vi "AlliGator Update Phasor Plot Image v2.vi"(5 "Image Control Refnum":T1 caption="Phasor Plot Display Refnum", 7 "Phasor Plot Color Scale":refnum<vi>, 8 "Error In":errorcluster, 9 "Phasor Plot Image Elements to Update":string[](array[string]), 10 "AlliGator Internal Variables DVR":refnum<data-value>, 11 "Phasor Plot Display Range Refnum":refnum<vi>) -> (0 "Error Out":errorcluster, 1 "Message":string, 2 "AlliGator Internal Variables DVR":refnum<data-value>)   [LabVIEW 2021, in "AlliGator Phasor Plot.lvlib"]
doc: "Updates the Phasor Plot image including its overlays."
uses:
  AlliGator Phasor Plot.lvlib
  Internal Variables/AlliGator Internal Variables v2.ctl
  <vilib>/vision/Image Controls.llb/IMAQ Image.ctl
  Internal Variables/AlliGator Gate Image Set.ctl
  Files/AlliGator FLI Dataset Type.ctl
  Files/AlliGator Data Series Type.ctl
  Dual-Channel Datasets/AlliGator Dataset Channel.ctl
  Settings/AlliGator Gate Arithmetic.ctl
  Source Image/AlliGator Displayed Image.ctl
  Image/Named ROI Description.ctl
  Phasor Graph/AlliGator Decay Metadata v3.ctl
  Decay Analysis/Decay Preprocessing/AlliGator Decay Background Subtraction Info.ctl
  Decay Analysis/Decay Preprocessing/AlliGator Baseline Subtraction Method.ctl
  Graphs/XY Graph/XY Graph Plot Shift Parameters.ctl
  Graphs/XY Graph/XY Graph Plot Shift Method.ctl
  Decay Analysis/Decay Preprocessing/AlliGator Decay Extrapolation Parameters.ctl
  Phasor/Calibration Phasor (m, phi).ctl
  Phasor/Phasor Reference Series.ctl
  Phasor/Phasor Calibration Map v2.ctl
  Phasor/Phasor (g, s).ctl
  Phasor Graph/AlliGator Raw Phasor Plot Data v5.ctl
  Phasor/Phasor Standard Deviation Options.ctl
  AlliGator Phasor Multi-Harmonic Data.ctl
  Phasor/Phasor Harmonic Data.ctl
  Decay Fit Parameter Map/AlliGator Decay Fit Options & Parameters v4.ctl
  Fits/IRF(X)PSED/Decay Fit Options v4.ctl
  Fits/Decay Convolution/Decay Model.ctl
  Fits/Residual Type.ctl
  Fits/IRF(X)PSED/Fit Weights Type v2.ctl
  Fits/Non-linear Fitting Method v2.ctl
  Fits/Fit Calculation Method.ctl
  Fits/Non-linear Fitting Algorithm.ctl
  Decay Analysis/Decay Fit/AlliGator Decay Fit Parameter Constraints 2.ctl
  Fits/IRF(X)PSED/Decay Fit Parameters In List.ctl
  Fits/IRF(X)PSED/MLE Baseline Offset Type.ctl
  Decay Analysis/Decay Preprocessing/AlliGator Decay Preprocessing Parameters.ctl
  Fits/IRF(X)PSED/Decay Fit Parameters & Derived Quantities List v2.ctl
  Fits/IRF(X)PSED/Decay Fit Result Constraint.ctl
  Decay Fit Parameter Map/AlliGator Parameter Maps Data.ctl
  Image/Image Control Refnum.ctl
  Globals, Variables, Constants/AlliGator Variables List.ctl
  a24687bc-c119-402d-9a1a-602e9bf75a15.vi
  Variant/Variant to Data/Variant to U16.vi
  Phasor Calibration/AlliGator Phasor Calibration.lvlib
  GUI/AlliGator GUI.lvlib
  Settings/AlliGator Settings.lvlib
  Time/Time.lvlib
  Globals, Variables, Constants/AlliGator Globals, Variables & Constants.lvlib
  Variant/Variant to Data/Variant to Data.lvlib
  Phasor/Phasor.lvlib
  7bec4d3f-1ec9-40da-bd4c-cfd082c5c359.vi
  Image/Image.lvlib
  Decay Analysis/Decay Preprocessing/AlliGator Decay Preprocessing.lvlib
  Graphs/XY Graph/XY Graph Add-Ons.lvlib
  Phasor Graph/AlliGator Phasor Graph.lvlib
  Files/AlliGator Files.lvlib
  Internal Variables/AlliGator Internal Variables.lvlib
  Source Image/AlliGator Source Image.lvlib
  Fits/Fits.lvlib
  Decay Analysis/Decay Fit/AlliGator Decay Fit.lvlib
  Dual-Channel Datasets/AlliGator Dual-Channel Datasets.lvlib
  Decay Fit Parameter Map/AlliGator Decay Fit Parameter Map.lvlib
panel:
  out "CPU (s)":dbl
  # "see the AlliGator License on the block diagram (Ctrl+E or Window:Show Block Diagram)"
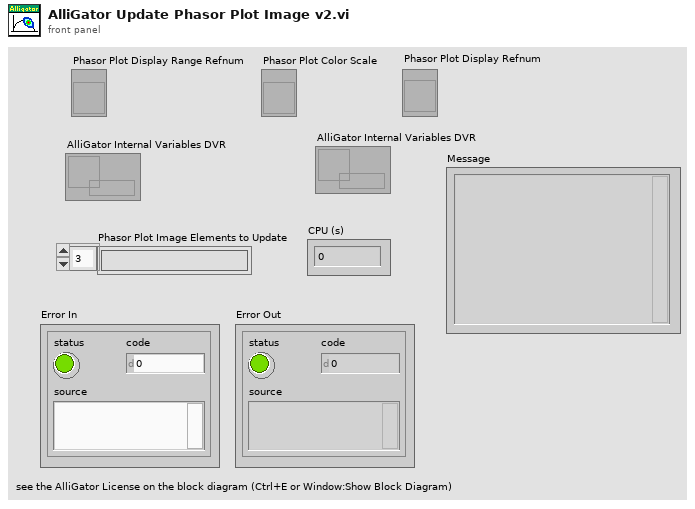
[diagram p1: front panel]
types:
  T1 = typedef "Image.lvlib/Image Control Refnum.ctl" = refnum<vi>
  T2 = typedef "AlliGator Globals, Variables & Constants.lvlib/AlliGator Variables List.ctl" = enum16{"---- GUI ----", "GUI:Initialization Status", "GUI:State Indicators Refnum", "GUI:Original AlliGator Menu Items", "GUI:Current Action Loop State", "GUI:Script in progress", "GUI:Playback", "GUI:Loop Playback", "GUI:Search ROI Used", "GUI:Search ROI", "Decay Graph Max Legend Size", "Intensity Graph Max Legend Size", "Decay Statistics Graph Max Legend Size", "Phasor Graph Max Legend Size", "Phasor Ratio Graph Max Legend Size", "Lifetime Graph Max Legend Size", "---- Files ----", "Files:Export Dataset Frames as Individual Files", "Files:Show Batch Export Help Balloons", "Files:Frames in Dataset", "Files:ptu File Frame Start Indices", "Files:Current Frame in Dataset", "Files:Current Frame Timestamp", "Files:Dataset Loaded", "Files:Dataset Metadata", "Files:Dataset Channel", "Files:Dataset Data Description", "Files:Background Dataset Metadata", "Files:Background Dataset Channel", "Files:Background Dataset Data Description", "Files:Background File Subtraction", "Files:Background File Path", "Files:Background File Pile-up Correction", "Files:Background File Pixel Well Capacity", "Files:Background File Scaling Factor", "Files:Current Dataset Load Settings", "Files:Dataset Path", "Files:ICCD-specific Information", "Files:Macrotime Gate Separation", "------ Python Plugins ------", "Python Plugins:Information", "Python Plugins:Python Session", "Python Plugins:Valid Python Session?", "---- Source Image ----", "Source Image:ROIs", "Source Image:Current ROI", "Source Image:ROI Event Refnum", "X_Source Image:Display Range", "X_Source Image:Palette Information", "X_Source Image:Type of Displayed Image", "X_Time Gate Slider", "Source Image:Palette List", "Source Image:Scale", "Source Image:ROI Overlay Color", "Source Image:Overlay to Erase", "Source Image:Is Displayed Image Accumulated", "Source Image:White Light Image Modified", "Source Image:Mask Image Modified", "---- Image Profile Window ----", "Image Profile:Window Event Refnum", "Image Profile:IntensityType", "Image Profile:Intensity Average Type", "Image Profile:Intensity-weighted SDV", "Image Profile:Box Profile Type", "Image Profile:Window Open", "Image Profile:Plotted Fit Parameter", "------ Phasor Graph -------", "Phasor Graph:Show Line", "---- Phasor Plot ---", "Phasor Plot:Parameters Changed", "Phasor Plot:FLI Dataset Modified since last Calculation", "Phasor Harmonics Data", "Selected Phasor Harmonics", "Phasor Harmonic Manager Event Refnum", "Phasor Plot:ROIs", "Phasor Plot:Current ROI", "Phasor Plot:ROI Event Refnum", "Phasor Plot:Image Reference Points", "Phasor Plot:Computed", "Phasor Plot:Palette Information", "Phasor Plot:Palette List", "Phasor Plot:Phasor Ratio Palette Information", "Phasor Plot:Phasor Ratio Palette List", "Phasor Plot:Image Scale", "Phasor Plot:Image Overlay to Erase", "Phasor Plot:Image Elements to Update", "Phasor Plot:Current Calculation Parameters", "Phasor Plot:Current Calibration Options", "Phasor Plot:Reset Cumulated Phasor Plot", "Phasor Plot:Reference 1", "Phasor Plot:Lifetime Reference 1", "Phasor Plot:Reference 1 Frequency", "Phasor Plot:Reference 2", "Phasor Plot:Lifetime Reference 2", "Phasor Plot:Reference 2 Frequency", "---- Decay Analysis ----", "Number of Selected Decays to Fit", "LS Fit Results", "LAR Fit Results", "BS Fit Results", "Last Decay Max - Min", "Best Fit Parameters", "Best Fit Parameter Names", "Actual Size X", "Actual Size Y", "Binning X", "Binning Y", "Actual # Gates", "Dataset Number", "Gates to...", "Gates Skipped", "Gates to keep", "Gate Step", "Gate Separation", "Reversed Gates", "Pile-up Correction", "Pixel Well Capacity", "Background Subtracted", "Background Subtraction Method", "Background Definition Range", "Background File (deprecated)", "Number of Dataset Accumulated", "Array of Accumulated Dataset Paths", "Do Averaged Datasets", "Destination File Path", "Process Plot Target", "Use 1/D as Phasor Frequency", "---- Decay Fit Parameter Map -----", "Decay Fit Parameter Map:Palette Information", "Decay Fit Parameter Map:Palette List", "Decay Fit Parameter Map:X Resolution", "Decay Fit Parameter Map:Y Resolution", "Decay Fit Parameter Map:Use Decay Fit Result Constraints", "Decay Fit Parameter Map:Decay Fit Result Constraints", "Decay Fit Parameter Map:Decay Fit Result Constraints Applied", "---- Parameter Map ----", "Parameter Map:Palette Information", "Parameter Map:Palette List", "------- Local Decay Window ---------", "Local Decay Graph Window:Event Refnum", "Local Decay Graph Window:Use normalized IRF for convolution", "----- Miscellaneous ----", "Misc:Skippable Dialog Windows Status"}
  T3 = typedef "AlliGator Internal Variables.lvlib/AlliGator Internal Variables v2.ctl" = cluster{"----------------------------- Images -----------------------------":u8, "Displayed Image":T4, "White Light Image":T4, "Mask Image":T4, "ROI Mask Image":T4, "Current Dataset Images 1":T5, "Background Dataset Images 1":T5, "Current Dataset Images 2":T5, "Background Dataset Images 2":T5, "Current Dataset Arithmetic Images":T5, "Accumulated Dataset Images 1":T5, "Accumulated Dataset Images 2":T5, "Accumulated Dataset Arithmetic Images":T5, "----------------------------- File Paths -----------------------------":u8, "Phasor Plot Image":T4, "Decay Fit Parameter Map Image":T4, "Parameter Map Image":T4, "Single Data Point Path":path, "White Light Image Path":path, "Mask Image Path":path, "Time-Series Folder":path, "[Time-Series Paths]":path[], "----------------------------- FLI Dataset -----------------------------":u8, "Current Dataset":i32, "Single Dataset Type":T6, "Current Folder":string, "AlliGator Data Series Type":T7, "# Datasets":i32, "Dual-Channel Dataset":bool, "Selected Channel Name":string, "Dataset Channel":T8, "Channel Arithmetic":T9, "Dual-Channel Background Dataset":bool, "Background Channel":T8, "Dual-Channel Accumulated Dataset":bool, "Start Time":dbl, "[Time-Series Timestamps]":dbl[], "[Intensity Corrections]":dbl[], "Time Series Script":bool, "Type of Displayed Image":T10, "Gate Image Slide":u16, "# Gates":i32, "ROIs":T11[], "----------------------------- Decays -----------------------------":u8, "ROI Decay":cluster{"t Array":dbl[], "I Array":dbl[]}, "Valid Decay":bool, "Decay  Metadata":T13, "Reference Decay Plot Name":string, "Reference Decay":cluster{"t Array":dbl[], "I Array":dbl[]}, "Decay Shift Plot":cluster{"Time Stamps":dbl[], "Decay Shifts":dbl[]}, "[Decays Max Values]":sgl[], "[Decays Min Values]":sgl[], "----------------------------- Calibration -----------------------------":u8, "Calibration Phasor":T19, "Calibration Phasor Series":T20, "Phasor Calibration Map":T21, "Calibration Map MD5 Digest":string, "----------------------------- Phasor Graph -----------------------------":u8, "Last Raw Phasor":T22, "Last Calibrated Phasor":T22, "Last Calibrated Phasor SDV":T22, "Phasor Graph:Phasor Plot":cluster{"g Array":dbl[], "s Array":dbl[]}, "Phasor Graph:Phasor SDV Plot":cluster{"g Array":dbl[], "s Array":dbl[]}, "[Phasor Graph:Raw Phasor Plots]":T23[], "Phasor Plot locked to Ref 1":i32, "[Phasor Plot(s) locked to Ref 1]":i32[], "[Phasor Plot(s) locked to Ref 2]":i32[], "[Pixel Phasors]":T22[], "----------------------------- Phasor Plot -----------------------------":u8, "[[Sum Image]]":dbl[][], "[[CSG Phasors]]":csg[][], "[[Valid Pixel?]]":bool[][], "[[Phasor Ratios]]":dbl[][], "[[Average Lifetimes]]":dbl[][], "Amplitude Weighted Average Lifetime":bool, "I/m/phi Dataset":cluster{"I/m/phi Dataset?":bool, "Base Frequency":dbl[unit], "Harmonic Orders":u8[]}, "Multi Phasor Plot Data":T25, "----------------------------- Decay Fit Parameter Map -----------------------------":u8, "Decay Fit Options & Parameters":T27, "Fit Options: Decay Preprocessing Parameters":T38, "Fit Options: Reference Decay":cluster{"t Array":dbl[], "I Array":dbl[]}, "Is Full Image Parameters Map":bool, "Is Single-Pixels Parameters Map":bool, "NLSF Parameters Map X Resolution":i32, "NLSF Parameters Map Y Resolution":i32, "[Single Decay Fit Parameters]":dbl[], "Fit Model":T29, "[[Multiple Decays Fit Parameters]]":dbl[][], "[[Multiple Decays Fit Parameter SDVs]]":dbl[][], "[[IRFs]]":dbl[][], "[ROI Descriptors]":T12[], "IRF Array Time Axis":dbl[], "Decay Array Time Axis":dbl[], "[Decay Fit Parameter Names]":T39[], "[Decay Sum]":dbl[], "Array of Decay Fit Result Constraints":T40[], "Selected ROIs Array":bool[], "----------------------------- Parameter Maps -----------------------------":u8, "[Map Set Names]":string[], "[Parameter Maps]":T41[], "[[User-defined Quantities]]":dbl[][], "User-defined Quantity":string}
  T4 = typedef "IMAQ Image.ctl" = refnum<image>
  T5 = typedef "AlliGator Internal Variables.lvlib/AlliGator Gate Image Set.ctl" = cluster{"SGL Gate Images":T4[], "SGL Sum Image":T4, "SGL Max Image":T4, "SGL Min Image":T4}
  T6 = typedef "AlliGator Files.lvlib/AlliGator FLI Dataset Type.ctl" = enum16{"HDF5 FLI Dataset", "Gate Image Folder", ".sdt FLI Dataset (Becker & Hickl)", ".ptu FLI Dataset (PicoQuant)", "SS1 FLI Dataset", "SS2 FLI Dataset", "I/m/phi Dataset", ".bin FLI Dataset (PicoQuant Binned)", ".bin FLI Dataset (Piccolo Binned)", ".mat FLI Dataset"}
  T7 = typedef "AlliGator Files.lvlib/AlliGator Data Series Type.ctl" = enum16{"Not a Supported Series", "Gate Images Folder Series", "SwissSPAD 2 Dataset Series", "B&H FLI Dataset Series", "PicoQuant PTU FLI Dataset Series", "PicoQuant BIN FLI Dataset Series", "Piccolo hist BIN FLI Dataset Series", "HDF5 FLI Dataset Series"}
  T8 = typedef "AlliGator Dual-Channel Datasets.lvlib/AlliGator Dataset Channel.ctl" = enum16{"G2", "INT"}
  T9 = typedef "AlliGator Settings.lvlib/AlliGator Gate Arithmetic.ctl" = enum16{"None", "INT-G2", "G2/INT*<INT>", "(1 - G2/INT)*<INT>"}
  T10 = typedef "AlliGator Source Image.lvlib/AlliGator Displayed Image.ctl" = enum16{"Single Gate", "Sum of All Gates", "Max of All Gates", "Min of All Gates", "-", "White Ligth Image", "Mask Image"}
  T11 = typedef "Image.lvlib/Named ROI Description.ctl" = cluster{"ROI Descriptor":T12, "ROI Name":string, "Overlay Color":u32}
  T12 = typedef "ROI Descriptor" = cluster{"Global Rectangle":i32[], "Contours":cluster{"ID":enum32{"External", "Internal"}, "Type":u32, "Coordinates":i32[]}[]}
  T13 = typedef "AlliGator Phasor Graph.lvlib/AlliGator Decay Metadata v3.ctl" = cluster{"ROI Descriptor":T12, "ROI Center":cluster{"X":i32, "Y":i32}, "Decay Background Subtraction Info":T14, "Decay Reverted":bool, "Decay Smoothened":bool, "Decay Straightened":bool, "Fitted Tau (Decay Straightening)":dbl, "Decay Shift Parameters":T16, "Decay Shifted":bool, "Decay Extrapolated":bool, "Decay Extrapolation Parameters":T18, "Decay Normalized":bool, "Fold Decay":bool, "# Folds":u32}
  T14 = typedef "AlliGator Decay Preprocessing.lvlib/AlliGator Decay Background Subtraction Info.ctl" = cluster{"Laser Period":dbl[unit], "Gate Duration":dbl[unit], "Baseline Subtraction Method":T15, "Background Definition Range":cluster{"Min Gate":dbl[unit], "Max Gate":dbl[unit]}, "Total Intensity w/o Bkgd Subtraction":dbl, "Bkgd-subtracted Intensity (exp)":dbl, "# Data Points":i32, "Background/Gate":dbl, "Fitted Lifetime":dbl[unit], "Bkgd-subtracted Intensity (theo)":dbl}
  T15 = typedef "AlliGator Decay Preprocessing.lvlib/AlliGator Baseline Subtraction Method.ctl" = enum16{"Mean", "Min", "Square Gated Single-Exponential", "File", "Constant"}
  T16 = typedef "XY Graph Add-Ons.lvlib/XY Graph Plot Shift Parameters.ctl" = cluster{"Type":T17, "Shift":dbl[unit], "Threshold":dbl, "Rotate":bool}
  T17 = typedef "XY Graph Add-Ons.lvlib/XY Graph Plot Shift Method.ctl" = enum16{"Default", "CFD", "Threshold", "Cross-Correlation"}
  T18 = typedef "AlliGator Decay Preprocessing.lvlib/AlliGator Decay Extrapolation Parameters.ctl" = cluster{"Additional Points":u32, "Head Fraction":dbl, "Fitted Tau":dbl, "Use Periodicity":bool, "Use Cursors":bool, "Tail Fraction":dbl}
  T19 = typedef "Phasor.lvlib/Calibration Phasor (m, phi).ctl" = cluster{"m":dbl, "phi":dbl, "Phasor Frequency":dbl[unit], "Reference Lifetime":dbl[unit]}
  T20 = typedef "Phasor.lvlib/Phasor Reference Series.ctl" = cluster{"m Array":dbl[], "phi Array":dbl[], "Phasor Frequency":dbl[unit], "Calibration Lifetime":dbl[unit]}
  T21 = typedef "Phasor.lvlib/Phasor Calibration Map v2.ctl" = cluster{"Phasor Frequency":dbl[unit], "Calibration Lifetime":dbl[unit], "ROI Centers":cluster{"X":i32, "Y":i32}[], "ROI Descriptors":T12[], "Map Resolution X":i32, "Map Resolution Y":i32, "z Array":cdb[]}
  T22 = typedef "Phasor.lvlib/Phasor (g, s).ctl" = cluster{"g":dbl, "s":dbl}
  T23 = typedef "AlliGator Phasor Graph.lvlib/AlliGator Raw Phasor Plot Data v5.ctl" = cluster{"Phasor Plot Name":string, "Raw Phasor Plot":T22[], "Phasor Frequency":dbl[unit], "[Decay Metadata]":T13[], "Raw Phasor Plot SDV":T22[], "Phasor SDV Options":T24, "[Calibration Phasor]":T19[], "Intensity Array":dbl[]}
  T24 = typedef "Phasor.lvlib/Phasor Standard Deviation Options.ctl" = cluster{"Compute Estimated SDV":bool, "# Replicas":u32, "Use Estimated Average Phasor":bool}
  T25 = typedef "AlliGator Phasor Plot.lvlib/AlliGator Phasor Multi-Harmonic Data.ctl" = cluster{"Base Frequency":dbl[unit], "# Harmonics":u8, "Harmonic Orders":u8[], "Phasor Plot Settings Checksum":u64, "Phasor Harmonic Data Array":T26[]}
  T26 = typedef "Phasor.lvlib/Phasor Harmonic Data.ctl" = cluster{"Phasor Harmonic Name":string, "Phasor Plot Settings Checksum":u64, "Phasor Frequency":dbl[unit], "Base Frequency":dbl[unit], "Harmonic Order":u8, "Phasor Plot Parameters":string, "Phasor Array [[CSG]]":csg[][], "Dataset File Path":path}
  T27 = typedef "AlliGator Decay Fit Parameter Map.lvlib/AlliGator Decay Fit Options & Parameters v4.ctl" = cluster{"SYNC Period":dbl[unit], "Fit Options":T28, "Fit Parameter Constraints":T35[], "MLE Baseline Offset":dbl, "MLE Baseline Offset Type":T37}
  T28 = typedef "Fits.lvlib/Decay Fit Options v4.ctl" = cluster{"Show Fit Residuals":bool, "Fit Model":T29, "Residual Type":T30, "Max Decay Percentile":dbl, "Min Decay Percentile":dbl, "Show Full Decay":bool, "Weights":T31, "Fitting Method":T32, "Compute Parameter Uncertainties":bool, "Periodic Boundaries":bool, "Model Calculation":T33, "Period":dbl[unit], "Termination Criteria":cluster{"Max Iterations":i32, "Max Function Calls":i32, "Max Time":dbl[unit], "Function Tolerance":dbl, "Parameter Tolerance":dbl, "Gradient Tolerance":dbl, "Min Lambda":dbl, "Max Lambda":dbl, "Initial Tick Count":u32}, "Offset Resolution":dbl[unit], "Use Local IRF":bool, "Fitting Algorithm":T34, "Show Confidence Interval ":bool, "Confidence Level":dbl}
  T29 = typedef "Fits.lvlib/Decay Model.ctl" = enum16{"1-Exponential", "2-Exponentials"}
  T30 = typedef "Fits.lvlib/Residual Type.ctl" = enum16{"Standard", "Normalized", "Reduced"}
  T31 = typedef "Fits.lvlib/Fit Weights Type v2.ctl" = enum16{"Unweighted", "1/Variance (Neyman)", "1/Variance (Pearson)", "Best of All"}
  T32 = typedef "Fits.lvlib/Non-linear Fitting Method v2.ctl" = enum16{"Least Square", "Least Absolute Residual", "Bisquare", "MLE", "-", "Best of All"}
  T33 = typedef "Fits.lvlib/Fit Calculation Method.ctl" = enum16{"Simulation", "Convolution", "Integration"}
  T34 = typedef "Fits.lvlib/Non-linear Fitting Algorithm.ctl" = enum16{"Levenberg-Marquardt", "Trust-Region Dogleg"}
  T35 = typedef "AlliGator Decay Fit.lvlib/AlliGator Decay Fit Parameter Constraints 2.ctl" = cluster{"Fit Parameter":T36, "Min Value":dbl, "Max Value":dbl, "Global":bool, "Used":bool}
  T36 = typedef "Fits.lvlib/Decay Fit Parameters In List.ctl" = enum16{"Offset", "Baseline", "A_1", "tau_1", "A_2", "tau_2"}
  T37 = typedef "Fits.lvlib/MLE Baseline Offset Type.ctl" = enum32{"Absolute", "Percentage"}
  T38 = typedef "AlliGator Decay Preprocessing.lvlib/AlliGator Decay Preprocessing Parameters.ctl" = cluster{"Background Subtraction":bool, "Straighten Decay":bool, "Reverse Gates":bool, "1-Normalized Decay":bool, "Smoothen Decay":bool, "Smoothing Parameter":dbl, "Shift Decay":bool, "Decay Shift Parameters":T16, "Extrapolate Decay":bool, "Additional Points":u32, "Head Fraction":dbl, "Pixel-Normalize Decay":bool, "Use Periodicity":bool, "Use Cursors":bool, "Tail Fraction":dbl, "Use Decay Pre-Processing":bool, "Fold Decay":bool, "# Folds":u32, "[0-1]-Normalized Decay":bool}
  T39 = typedef "Fits.lvlib/Decay Fit Parameters & Derived Quantities List v2.ctl" = enum16{"Offset", "Baseline", "A_1", "tau_1", "A_2", "tau_2", "<tau>_a", "f1_a", "f2_a", "<tau>_i", "f1_i", "f2_i", "-", "R^2", "Chi^2"}
  T40 = typedef "Fits.lvlib/Decay Fit Result Constraint.ctl" = cluster{"Fit Parameter":enum16{"Offset", "Baseline", "A_1", "tau_1", "A_2", "tau_2", "<tau>_a", "f1_a", "f2_a", "<tau>_i", "f1_i", "f2_i", "-", "R^2", "Chi^2", "Max Relative Residual", "<Residual ACF>", "Residual ACF SDV", "tau_2/tau_1"}, "Min Value":dbl, "Max Value":dbl, "Use Constraint":bool}
  T41 = typedef "AlliGator Decay Fit Parameter Map.lvlib/AlliGator Parameter Maps Data.ctl" = cluster{"Map Set Name":string, "[Parameter Names]":string[], "[[Parameters]]":dbl[][], "[[Parameter SDVs]]":dbl[][], "Decay Array Time Axis":dbl[], "[[IRFs]]":dbl[][], "IRF Array Time Axis":dbl[], "X Resolution":i32, "Y Resolution":i32, "Intensity Array":dbl[]}
  T42 = typedef "Phasor.lvlib/Phasor Calibration Type.ctl" = enum16{"None", "Single Phasor", "Phasor Series", "Phasor Map"}
  T43 = cluster{"Use Backup Calibration if needed?":bool, "Calibration Type":T42}
  T44 = typedef "AlliGator Phasor Calibration.lvlib/AlliGator Phasor Calibration Options.ctl" = cluster{"Phasor Frequency":dbl[unit], "Phasor Calibration":cluster{"Calibration Lifetime":dbl[unit], "Calibration Type":T42, "Calibration Map Algorithm":T45, "Use Backup Calibration if needed":bool, "Backup Calibration Type":enum16{"Single Calibration", "Nearest Valid Calibration"}}}
  T45 = typedef "AlliGator Phasor Calibration.lvlib/AlliGator Calibration Map Algorithm.ctl" = enum16{"Simple Search", "Min Distance"}
  T46 = typedef "AlliGator Phasor Plot.lvlib/AlliGator Phasor Plot Parameters v2.ctl" = cluster{"Phasor Frequency":dbl[unit], "Decay Preprocessing Options & Parameters":T47, "FLI Dataset Modified":bool, "Source Image Settings":cluster{"Low Count Pixels Rejection Options":T49, "High Count Pixels Rejection Options":T50}, "Data Information":cluster{"Gate Width":dbl[unit], "Gate Separation":dbl[unit], "Step (Gate Separation)":i32, "Laser Period":dbl[unit], "SYNC Period":dbl[unit], "Channel Name":u16, "Channel Arithmetic":T9, "Pile-up Correction":bool, "Pixel Well Capacity":u32, "Dataset Scaling Factor":dbl}, "Phasor Plot":cluster{"Phasor Plot Smoothing Options":T51, "Phasor Plot Size":T54, "Selected Image ROI(s)":bool, "All Image ROIs":bool, "Selected Source Image ROI":i32, "Source Image ROIs":T11[]}}
  T47 = typedef "AlliGator Decay Preprocessing.lvlib/AlliGator Decay Preprocessing Options.ctl" = cluster{"Background Subtraction Parameters":T48, "Decay Preprocessing Parameters":T38, "Preprocessing Steps Order":string[]}
  T48 = typedef "AlliGator Decay Preprocessing.lvlib/AlliGator Background Subtraction Parameters.ctl" = cluster{"Background Definition Range":cluster{"Min Gate":dbl[unit], "Max Gate":dbl[unit]}, "Baseline Subtraction Method":T15, "Background Subtraction?":bool, "Background File":path, "Background Constant":dbl, "Background Scaling Factor":dbl, "Background Pile-up Correction":bool, "Background Pixel Well Capacity":u32}
  T49 = typedef "AlliGator Settings.lvlib/AlliGator Low Count Pixels Rejection Options.ctl" = cluster{"Background Low Threshold Factor":dbl, "Fixed Low Background Threshold":dbl, "Reject Low Count Pixels":bool, "Low Percentile":dbl}
  T50 = typedef "AlliGator Settings.lvlib/AlliGator High Count Pixels Rejection Options.ctl" = cluster{"Background High Threshold Factor":dbl, "Fixed High Background Threshold":dbl, "Reject High Count Pixels":bool, "High Percentile":dbl}
  T51 = typedef "AlliGator Phasor Plot.lvlib/AlliGator Phasor Plot Smoothing Options.ctl" = cluster{"Use Phasor Plot Smoothing":bool, "Kernel Type":T52, "Bin":i32, "Algorithm":T53}
  T52 = typedef "Arrays.lvlib/Kernel Type.ctl" = enum16{"Uniform", "Bilinear", "Gaussian"}
  T53 = typedef "Arrays.lvlib/Smoothing Algorithm.ctl" = enum16{"Rapid", "Thorough"}
  T54 = typedef "AlliGator Phasor Plot.lvlib/AlliGator Phasor Plot Size.ctl" = cluster{"H":i32, "V":i32, "Margin":dbl}
  T55 = typedef "Phasor.lvlib/Phasor Calibration Map Characteristics.ctl" = cluster{"Phasor Frequency":dbl[unit], "Calibration Lifetime":dbl[unit], "Map Resolution X":i32, "Map Resolution Y":i32, "Empty Map":bool}
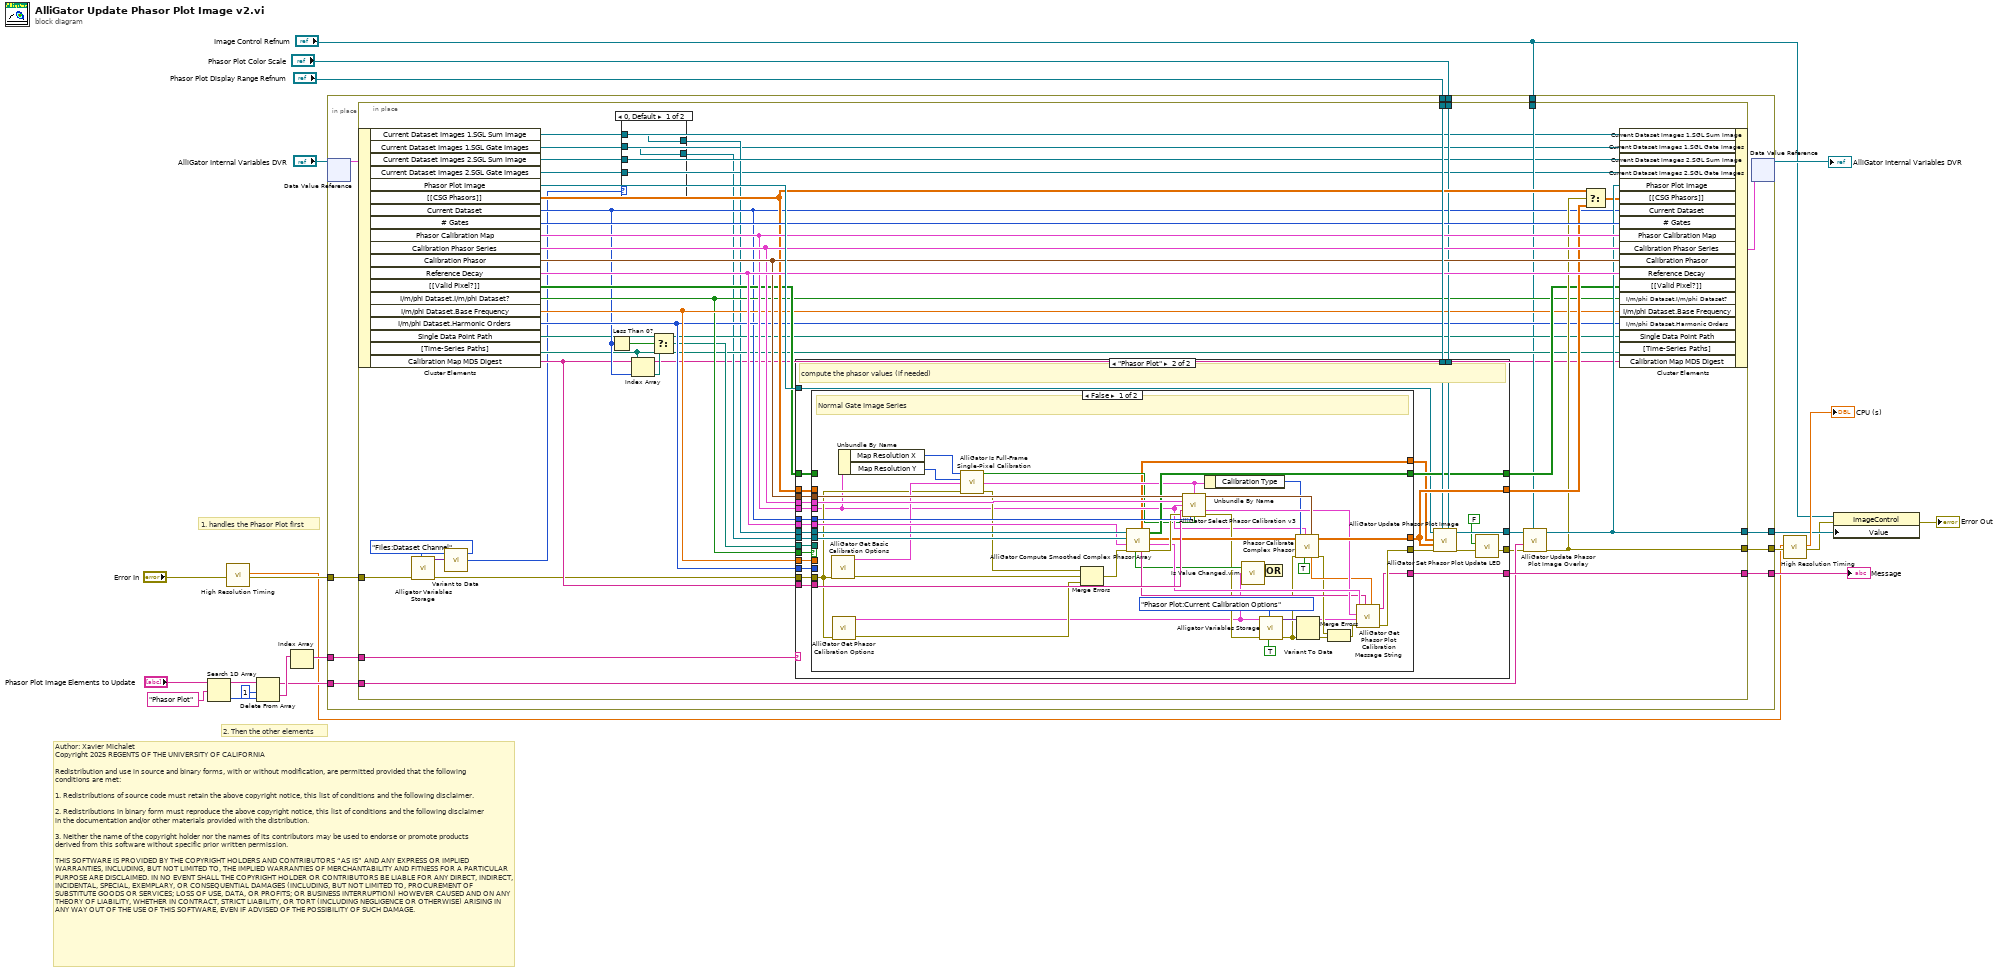
[diagram p0: block diagram]
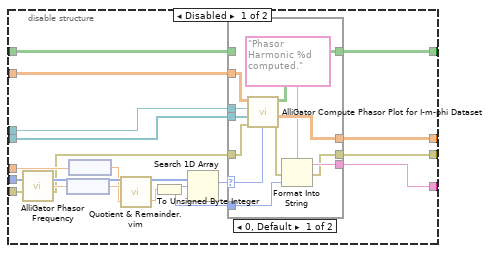
[diagram p4: hidden frame]
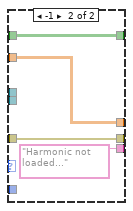
[diagram p5: hidden frame]
diagram:
  # "Author: Xavier Michalet\nCopyright 2025 REGENTS OF THE UNIVERSITY OF CALIFORNIA\n\nRedistribution and use in source and binary forms, with or without modification, are permitted provided that the following conditions are met:\n\n1. Redistributions of source code must retain the above copyright notice, this list of conditions and the following disclaimer.\n\n2. Redistributions in binary form must reproduce the above copyright notice, this list of conditions and the following disclaimer in the documentation and/or other materials provided with the distribution.\n\n3. Neither the name of the copyright holder nor the names of its contributors may be used to endorse or promote products derived from this software without specific prior written permission.\n\nTHIS SOFTWARE IS PROVIDED BY THE COPYRIGHT HOLDERS AND CONTRIBUTORS “AS IS” AND ANY EXPRESS OR IMPLIED WARRANTIES, INCLUDING, BUT NOT LIMITED TO, THE IMPLIED WARRANTIES OF MERCHANTABILITY AND FITNESS FOR A PARTICULAR PURPOSE ARE DISCLAIMED. IN NO EVENT SHALL THE COPYRIGHT HOLDER OR CONTRIBUTORS BE LIABLE FOR ANY DIRECT, INDIRECT, INCIDENTAL, SPECIAL, EXEMPLARY, OR CONSEQUENTIAL DAMAGES (INCLUDING, BUT NOT LIMITED TO, PROCUREMENT OF SUBSTITUTE GOODS OR SERVICES; LOSS OF USE, DATA, OR PROFITS; OR BUSINESS INTERRUPTION) HOWEVER CAUSED AND ON ANY THEORY OF LIABILITY, WHETHER IN CONTRACT, STRICT LIABILITY, OR TORT (INCLUDING NEGLIGENCE OR OTHERWISE) ARISING IN ANY WAY OUT OF THE USE OF THIS SOFTWARE, EVEN IF ADVISED OF THE POSSIBILITY OF SUCH DAMAGE."
  # "2. Then the other elements"
  # "1. handles the Phasor Plot first"
  n1 = Search 1D Array(1D array="Phasor Plot Image Elements to Update", element="Phasor Plot") -> (index of element=w19:i32)  [unwired: 1 in]
  n2 = call "High Resolution Timing.vi"("Error In"="Error In") -> ("elapsed (relative) seconds"=w6:dbl, "Error Out"=w7:errorcluster)  [unwired: 16 in, 1 out]
  n3 = Delete From Array(array="Phasor Plot Image Elements to Update", length=1, index=w19) -> (deleted portion=w17:string[], array with subset deleted=w14:string[])
  n4 = Index Array(array=w17) -> (element=w16:string)  [unwired: 1 in]
  n5 = in-place {
    in-place-border: [w32] -> w21
    in-place-border: w16 -> [w31]
    in-place-border: w7 -> [w30]
    in-place-border: [w29] -> w4
    in-place-border: [w28] -> w15
    in-place-border: w14 -> [w27]
    in-place-border: "Phasor Plot Display Range Refnum" -> [w24]
    in-place-border: "Phasor Plot Color Scale" -> [w23]
    in-place-border: "Image Control Refnum" -> [w22]
    n6 = in-place-dvr #1("AlliGator Internal Variables DVR") -> (w26:T3)  [unwired: 1 out]
    n7 = in-place {
      in-place-border: [w74] -> w32
      in-place-border: w31 -> [w73]
      in-place-border: w30 -> [w35]
      in-place-border: [w64] -> w29
      in-place-border: [w60] -> w28
      in-place-border: w27 -> [w72]
      in-place-border: w24 -> [w70]
      in-place-border: w23 -> [w59]
      in-place-border: w22 -> [w45]
      n8 = in-place-cluster #2(w26) -> ("Current Dataset Images 1.SGL Sum Image"=w44:T4, "Current Dataset Images 1.SGL Gate Images"=w41:T4[], "Current Dataset Images 2.SGL Sum Image"=w43:T4, "Current Dataset Images 2.SGL Gate Images"=w40:T4[], "Phasor Plot Image"=w71:T4, "[[CSG Phasors]]"=w61:csg[][], "Current Dataset"=w50:i32, "# Gates"=w65:i32, "Phasor Calibration Map"=w66:T21, "Calibration Phasor Series"=w67:T20, "Calibration Phasor"=w68:T19, "Reference Decay"=w69:cluster{"t Array":dbl[], "I Array":dbl[]}, "[[Valid Pixel?]]"=w58:bool[][], "I/m/phi Dataset.I/m/phi Dataset?"=w53:bool, "I/m/phi Dataset.Base Frequency"=w54:dbl[unit], "I/m/phi Dataset.Harmonic Orders"=w52:u8[], "Single Data Point Path"=w47:path, "[Time-Series Paths]"=w46:path[], "Calibration Map MD5 Digest"=w38:string)
      n9 = call "Alligator Variables Storage.vi"("AlliGator Variable"=AlliGator_Variables_List."Files:Dataset Channel" ("Alligator Variable"), "Error In"=w35) -> ("Error Out"=w34:errorcluster, "Data out"=w36:variant)  [unwired: 7 in, 1 out]
      n10 = call-poly "Variant to Data.vi"("Variant"=w36) -> ("U16 Value"=w33:u16)  [unwired: 8 in]
      n11 = Less Than 0?(x=w50) -> (x < 0?=w51:bool)
      n12 = case shown="0, Default" w33 {
        tunnel: [w197 w199] -> w42
        tunnel: w43 -> [_ w199]
        tunnel: [w196 w198] -> w39
        tunnel: w40 -> [_ w198]
        tunnel: w44 -> [w197 _]
        tunnel: w41 -> [w196 _]
        frame 0, Default {
        }
        frame 1 {
        }
      }
      n13 = Index Array(array=w46, index=w50) -> (element=w49:path)
      n14 = Select(t=w47, s=w51, f=w49) -> (s? t:f=w48:path)
      n15 = case shown="\"Phasor Plot\"" w73 {
        tunnel: w42 -> [_ w105]
        tunnel: [w76 w100] -> w63
        tunnel: w39 -> [_ w104]
        tunnel: [_ w101] -> w74
        tunnel: [w77 w90] -> w55
        tunnel: w71 -> [w78 w81]
        tunnel: [w78 w103] -> w56
        tunnel: w34 -> [w77 w96]
        tunnel: w61 -> [w76 w83]
        tunnel: w70 -> [_ w99]
        tunnel: w68 -> [_ w98]
        tunnel: w67 -> [_ w97]
        tunnel: w66 -> [_ w94]
        tunnel: w50 -> [_ w95]
        tunnel: w69 -> [_ w93]
        tunnel: w59 -> [_ w89]
        tunnel: [w75 w88] -> w57
        tunnel: w58 -> [w75 w84]
        tunnel: w53 -> [_ w87]
        tunnel: w54 -> [_ w86]
        tunnel: w52 -> [_ w85]
        tunnel: w48 -> [_ w82]
        tunnel: w38 -> [_ w80]
        frame "", Default {
          # "keep the current phasor values"
        }
        frame "Phasor Plot" {
          # "compute the phasor values (if needed)"
          n16 = case shown="False" w87 {
            tunnel: w105 -> [w148 w149]
            tunnel: w104 -> [w147 w152]
            tunnel: [w146 w153] -> w102
            tunnel: [w145 w155] -> w101
            tunnel: [w144 w156] -> w100
            tunnel: w98 -> [w143 _]
            tunnel: w97 -> [w142 _]
            tunnel: w96 -> [w112 w154]
            tunnel: w95 -> [w141 _]
            tunnel: w94 -> [w110 _]
            tunnel: w93 -> [w140 _]
            tunnel: [w139 w150] -> w88
            tunnel: w86 -> [_ w158]
            tunnel: w85 -> [_ w159]
            tunnel: w84 -> [_ w151]
            tunnel: w83 -> [_ w157]
            tunnel: w82 -> [_ _]
            tunnel: w80 -> [w138 _]
            tunnel: [w106 _] -> w79
            frame False {
              # "Normal Gate Image Series"
              n17 = call "AlliGator Get Basic Calibration Options.vi"("error in (no error)"=w112) -> ("error out"=w115:errorcluster, "Basic Calibration Options"=w114:T43)  [unwired: 9 in]
              n18 = call "AlliGator Get Phasor Calibration Options.vi"("Error In"=w112) -> ("Error Out"=w119:errorcluster, "Phasor Calibration Options"=w117:T44)  [unwired: 8 in, 1 out]
              n19 = Unbundle By Name(w110) -> ("Map Resolution X"=w109:i32, "Map Resolution Y"=w108:i32)
              n20 = call "AlliGator Is Full-Frame Single-Pixel Calibration.vi"("error in (no error)"=w112, "Map Resolution Y"=w108, "Map Resolution X"=w109) -> ("error out"=w111:errorcluster, "Full-Frame Single-Pixel Calibration?"=w107:bool)  [unwired: 7 in]
              n21 = Merge Errors(w111, w115, w119) -> (w116:errorcluster)
              n22 = call "AlliGator Compute Smoothed Complex Phasor Array.vi"("error in (no error)"=w116, "Time-Gated Reference Decay"=w140, "Image Array"=w147, "Sum Image"=w148) -> ("error out"=w137:errorcluster, "Phasor Plot Parameters"=w131:T46, "Corrected Complex Phasor Array out (VxH)"=w136:csg[][], "Valid Pixel?"=w139:bool[][], "Message"=w129:string, "Pre-processed Sum Image (V x H)"=w106:sgl[][], "Phasor Array updated"=w126:bool)  [unwired: 1 in]
              n23 = call "AlliGator Select Phasor Calibration v3.vi"("Calibration Phasor"=w143, "Basic Calibration Options"=w114, "Calibration Phasor Series"=w142, "Phasor Calibration Map"=w110, "Calibration Map MD5 Digest"=w138, "Error In"=w137, "Current Data Set (-1: single)"=w141, "Full-Frame Single-Pixel Calibration?"=w107) -> ("Calibration Phasor"=w135:T19, "Phasor Calibration Map Characteristics"=w130:T55, "Error Out"=w118:errorcluster)  [unwired: 5 in]
              n24 = Unbundle By Name(w114) -> ("Calibration Type"=w113:T42)
              n25 = call "Is Value Changed.vim"("value"=w117) -> ("changed or first call?"=w134:bool)
              n26 = call "Alligator Variables Storage.vi"("Get(F)/Set"=TRUE, "AlliGator Variable"=AlliGator_Variables_List."Phasor Plot:Current Calibration Options" ("Alligator Variable"), "Error In"=w118, "Data in"=w117) -> ("Error Out"=w123:errorcluster, "Data out"=w125:variant)  [unwired: 5 in, 1 out]
              n27 = Compound Arithmetic op=OR(w126, w134) -> ()  [unwired: 1 out]
              n28 = call "Phasor Calibrate Complex Phasor.vi"("Calibration Phasor"=w135, "Force Calibration (T)"=TRUE, "Phasor Calibration Map"=w110, "Error In"=w123, "Calibration Type Used"=w113, "Complex Phasor Array (VxH)"=w136) -> ("Error Out"=w127:errorcluster, "Corrected Complex Phasor Array (VxH)"=w144:csg[][], "CPU (s)"=w128:dbl)  [unwired: 3 in]
              n29 = Variant To Data(error in=w123, Variant=w125) -> (data=w124:T44, error out=w121:errorcluster)  [unwired: 1 in]
              n30 = Merge Errors(w127, w121) -> (w122:errorcluster)
              n31 = call "AlliGator Get Phasor Plot Calibration Message String.vi"("Calibration CPU (s)"=w128, "Message in"=w129, "error in (no error)"=w122, "AlliGator Phasor Calibration Options"=w124, "Phasor Calibration Map Characteristics"=w130, "Phasor Plot Parameters"=w131) -> ("error out"=w146:errorcluster, "Message out"=w145:string)  [unwired: 4 in]
            }
            frame True {
              # "I/m/phi Dataset"
              n32 = disable-structure shown="Enabled" {
                disable-tunnel: w159 -> [w173 _]
                disable-tunnel: w158 -> [w172 _]
                disable-tunnel: w157 -> [w170 w194]
                disable-tunnel: [w169 w194] -> w156
                disable-tunnel: [w168 _] -> w155
                disable-tunnel: w154 -> [w167 w193]
                disable-tunnel: [w166 w193] -> w153
                disable-tunnel: w152 -> [w165 _]
                disable-tunnel: w151 -> [w163 w195]
                disable-tunnel: [w162 w195] -> w150
                disable-tunnel: w149 -> [w161 _]
                frame Disabled {
                  n33 = call "AlliGator Phasor Frequency.vi"() -> ("Phasor Frequency"=w176:dbl[unit])
                  n34 = node(w176) -> (w175:dbl)
                  n35 = node(w172) -> (w160:dbl)
                  n36 = call "Quotient & Remainder.vim"("y"=w160, "x"=w175) -> ("E(x/y)"=w174:dbl)  [unwired: 1 out]
                  n37 = To Unsigned Byte Integer(number=w174) -> (unsigned 8bit integer=w164:u8)
                  n38 = Search 1D Array(1D array=w173, element=w164) -> (index of element=w171:i32)  [unwired: 1 in]
                  n39 = case shown="0, Default" w171 {
                    selector: w171 -> [w185 _]
                    tunnel: w170 -> [w186 w192]
                    tunnel: [w180 w192] -> w169
                    tunnel: [w184 "Harmonic not loaded..." ("Message")] -> w168
                    tunnel: w167 -> [w188 w190]
                    tunnel: [w182 w190] -> w166
                    tunnel: w165 -> [w187 _]
                    tunnel: w164 -> [w181 _]
                    tunnel: w163 -> [_ w189]
                    tunnel: [w179 w189] -> w162
                    tunnel: w161 -> [w178 _]
                    frame 0, Default {
                      n40 = call "AlliGator Compute Phasor Plot for I-m-phi Dataset.vi"("Harmonic index"=w185, "error in (no error)"=w188, "Image Array"=w187, "Sum Image"=w178, "[[CSG]] Phasor Array in"=w186) -> ("error out"=w183:errorcluster, "[[CSG]] Phasor Array out"=w180:csg[][], "Valid Pixel?"=w179:bool[][])  [unwired: 4 in]
                      n41 = Format Into String(format string="Phasor Harmonic %d computed.", error in=w183, w181) -> (resulting string=w184:string, error out=w182:errorcluster)  [unwired: 1 in]
                    }
                    frame -1 {
                    }
                  }
                }
                frame Enabled {
                }
              }
            }
          }
          n42 = call "AlliGator Update Phasor Plot Image.vi"("Phasor Plot Color Scale"=w89, "Phasor Plot Display Range Refnum"=w99, "error in (no error)"=w102, "Corrected Complex Phasor Array"=w100, "Pre-processed Sum Image (V x H)"=w79, "Phasor Plot Image in"=w81) -> ("error out"=w91:errorcluster, "Phasor Plot Image out"=w103:T4)  [unwired: 3 in, 1 out]
          n43 = call "AlliGator Set Phasor Plot Update LED.vi"("error in (no error)"=w91, "Off/On"=FALSE) -> ("error out"=w90:errorcluster)  [unwired: 9 in]
        }
      }
      n44 = call "AlliGator Update Phasor Plot Image Overlay.vi"("Image Control Refnum"=w45, "error in (no error)"=w55, "Overlay List"=w72, "Phasor Plot Image in"=w56) -> ("error out"=w60:errorcluster, "Phasor Plot Image out"=w64:T4)  [unwired: 6 in]
      n45 = Select(t=w61, s=w60, f=w63) -> (s? t:f=w62:csg[][])
      n46 = in-place-cluster #2("Current Dataset Images 1.SGL Sum Image"=w44, "Current Dataset Images 1.SGL Gate Images"=w41, "Current Dataset Images 2.SGL Sum Image"=w43, "Current Dataset Images 2.SGL Gate Images"=w40, "Phasor Plot Image"=w64, "[[CSG Phasors]]"=w62, "Current Dataset"=w50, "# Gates"=w65, "Phasor Calibration Map"=w66, "Calibration Phasor Series"=w67, "Calibration Phasor"=w68, "Reference Decay"=w69, "[[Valid Pixel?]]"=w57, "I/m/phi Dataset.I/m/phi Dataset?"=w53, "I/m/phi Dataset.Base Frequency"=w54, "I/m/phi Dataset.Harmonic Orders"=w52, "Single Data Point Path"=w47, "[Time-Series Paths]"=w46, "Calibration Map MD5 Digest"=w38) -> (w25:T3)
    }
    n47 = in-place-dvr #1(w25) -> (→"AlliGator Internal Variables DVR":refnum<data-value>)  [unwired: 1 out]
  }
  "Message" <- w21
  n48 = call "High Resolution Timing.vi"("relative seconds (NaN)"=w6, "Error In"=w15) -> ("elapsed (relative) seconds"=→"CPU (s)":dbl, "Error Out"=w3:errorcluster)  [unwired: 15 in, 1 out]
  n49 = property class="ImageControl"(reference="Image Control Refnum", error in=w3, "Value"=w4) -> (error out=→"Error Out":errorcluster)  [unwired: 1 out]
